vi "Laser Rough Cutting.vi"(0 "configuration file path":path caption="配置文件的路径", 1 "rough cutting msic":T1) -> ()   [LabVIEW 2014]
uses:
  Ctl.xio/rough cutting msic ctl.ctl
  SubVIS.xio/DataSocket/DataSocket_Tags.ctl
  Ctl.xio/part type.ctl
  SubVIS.xio/DataSocket/Write PLC Vars/Write String Var in.vi
  <vilib>/Utility/file.llb/Read From Spreadsheet File (string).vi
  SubVIS.xio/DataSocket/Write PLC Vars/Write Bool Var in.vi
  SubVIS.xio/DataSocket/Read PLC Vars/Read String Var.vi
  SubVIS.xio/DataSocket/Write PLC Vars/Write Dbl Var in.vi
  SubVIS.xio/DataSocket/Read PLC Vars/Read Bool Var.vi
  SubVIS.xio/DataSocket/Read PLC Vars/Read U32 Var.vi
panel:
  in  "SQL information":string
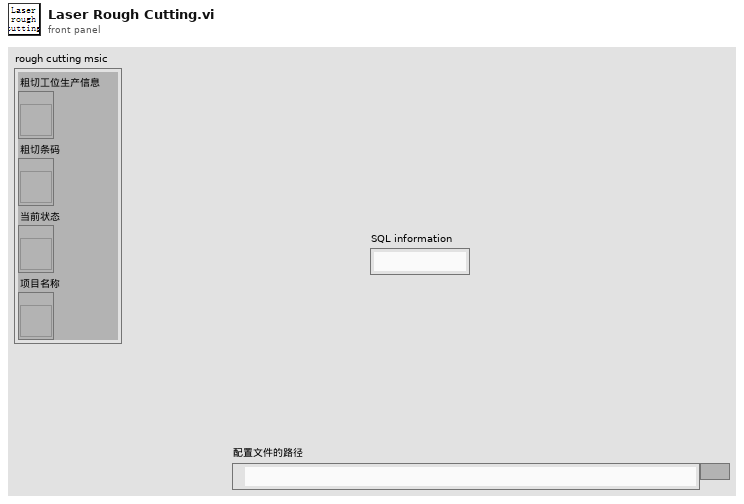
[diagram p1: front panel]
types:
  T1 = cluster{"粗切工位生产信息":refnum<vi>, "粗切条码":refnum<vi>, "当前状态":refnum<vi>, "项目名称":refnum<vi>}
  T2 = typedef "rough cutting msic ctl.ctl" = cluster{"configuration file path":path, "DsOut":T3[], "scanner coms or ip":string, "BarCode":string, "scanner resource name out":refnum<visa-resource-name>, "Hopper car information":cluster{"Hopper car code":string, "Hopper car No":string, "plate No":string}, "pallet.produced number":i32, "SQL information":string, "Database":string[], "Serial number":i32, "database path":path, "rough cutting msic":cluster{"粗切工位生产信息":refnum<vi>, "粗切条码":refnum<vi>, "当前状态":refnum<vi>, "项目名称":refnum<vi>}, "part type":T4, "scanner ip ID":refnum<k5>, "Number of scans ":u8}
  T3 = typedef "DataSocket_Tags.ctl" = cluster{"Ds ID":refnum<k13>, "Tag":string}
  T4 = typedef "part type.ctl" = cluster{"项目号":string, "物料代码":string, "零件号":string, "供应商编码":string, "产线编码":string, "客户代码":string, "颜色代码":string, "托盘上限":i32, "加热温度":string, "加热时长":string, "EOL Stations":string}
  T5 = cluster{"Hopper car code":string, "Hopper car No":string, "plate No":string}
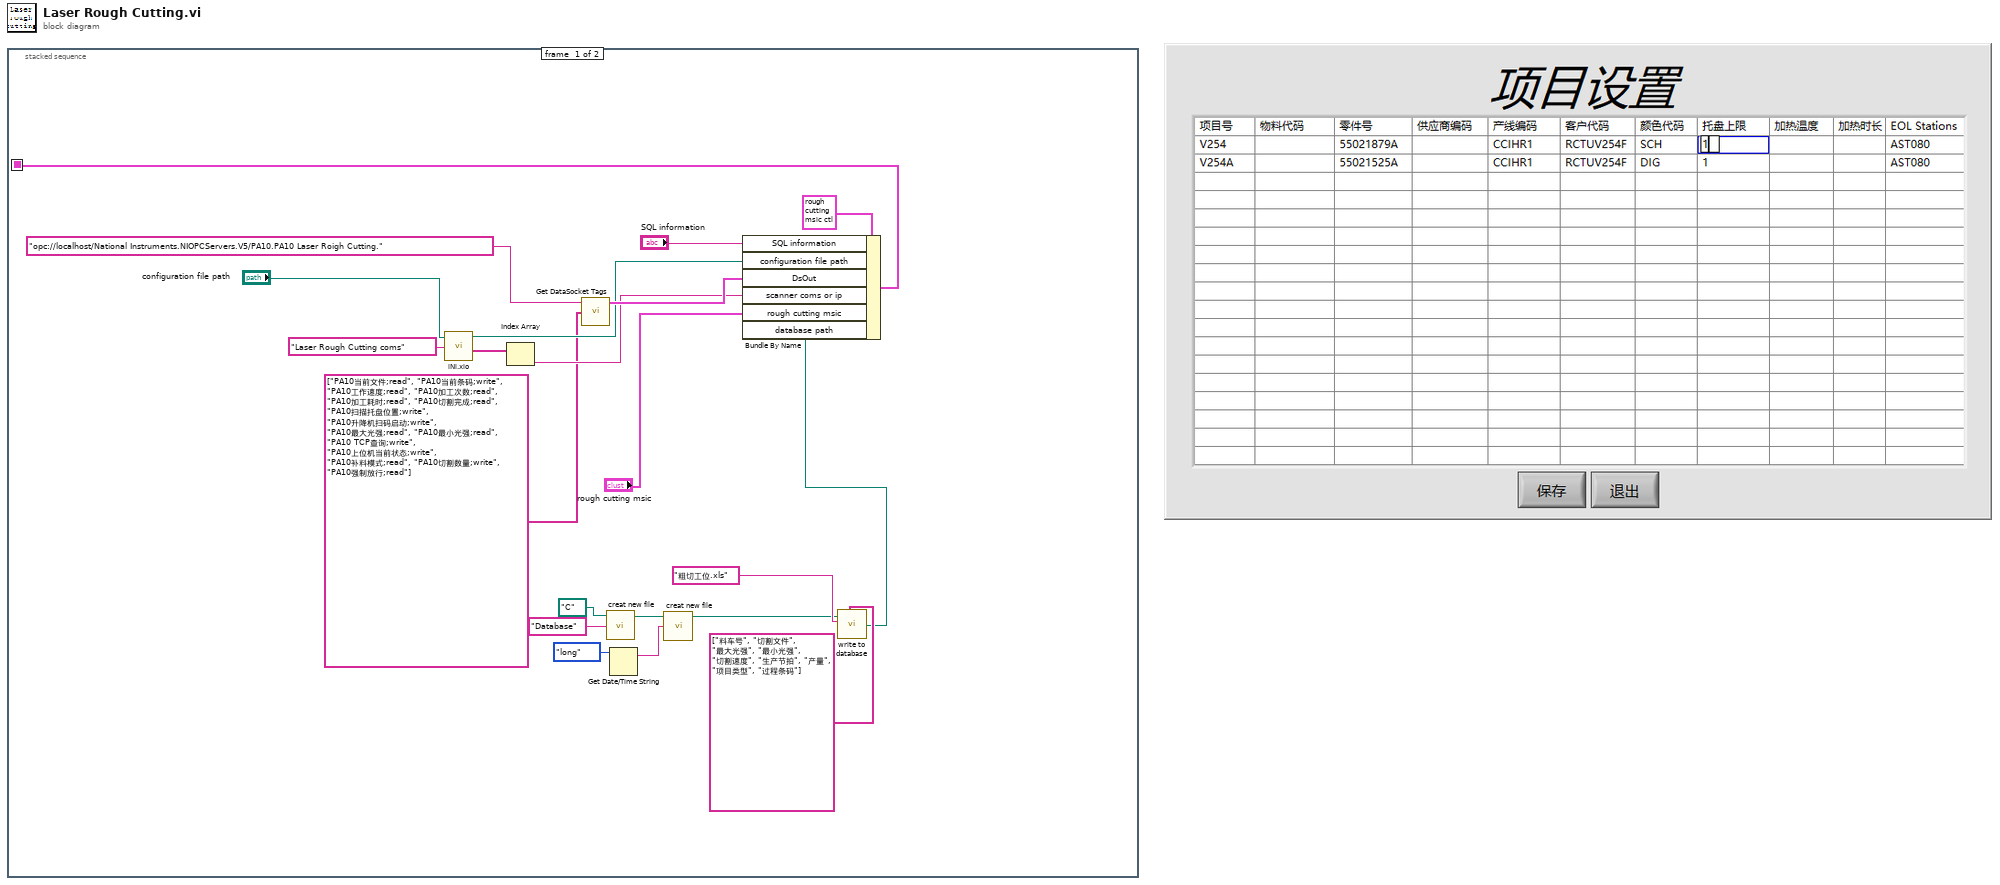
[diagram p0: block diagram]
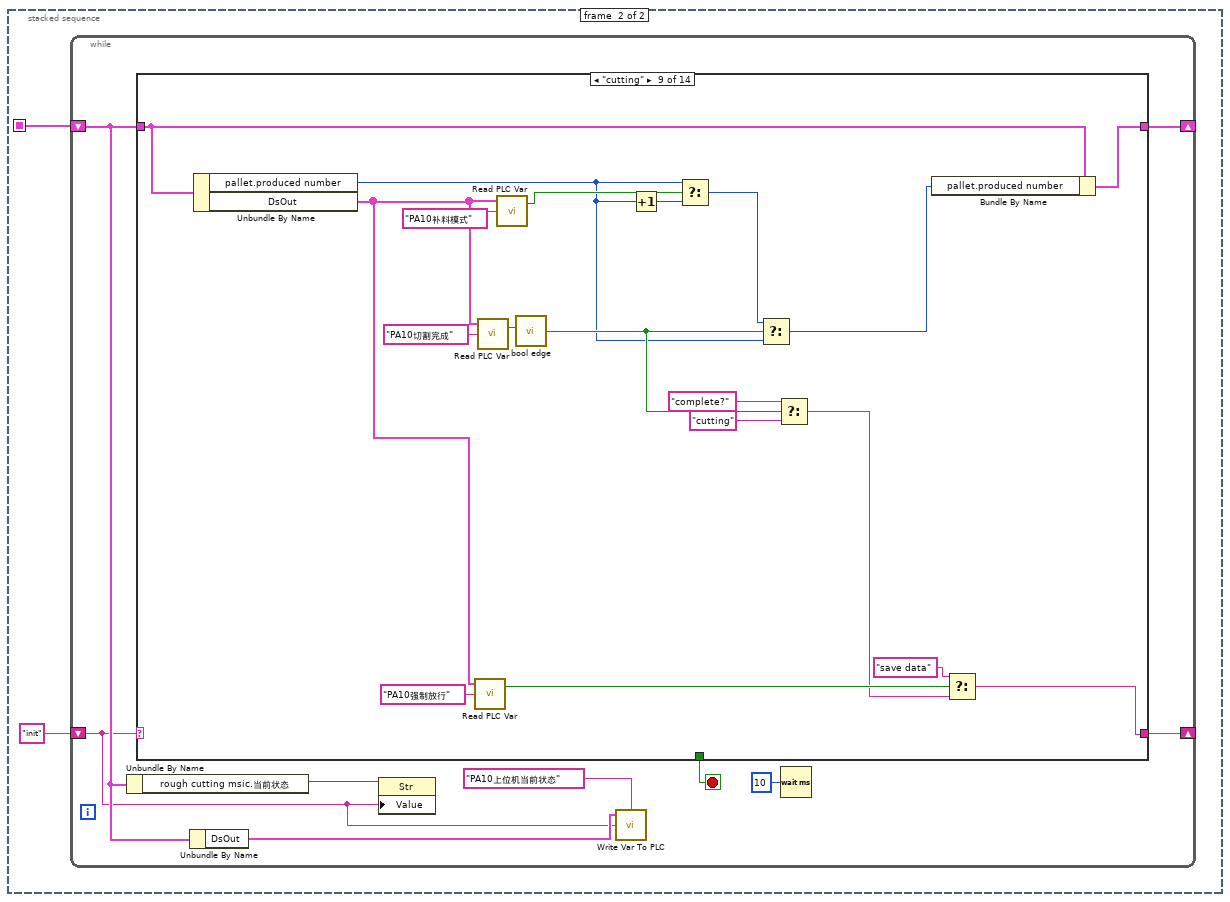
[diagram p2: hidden frame]
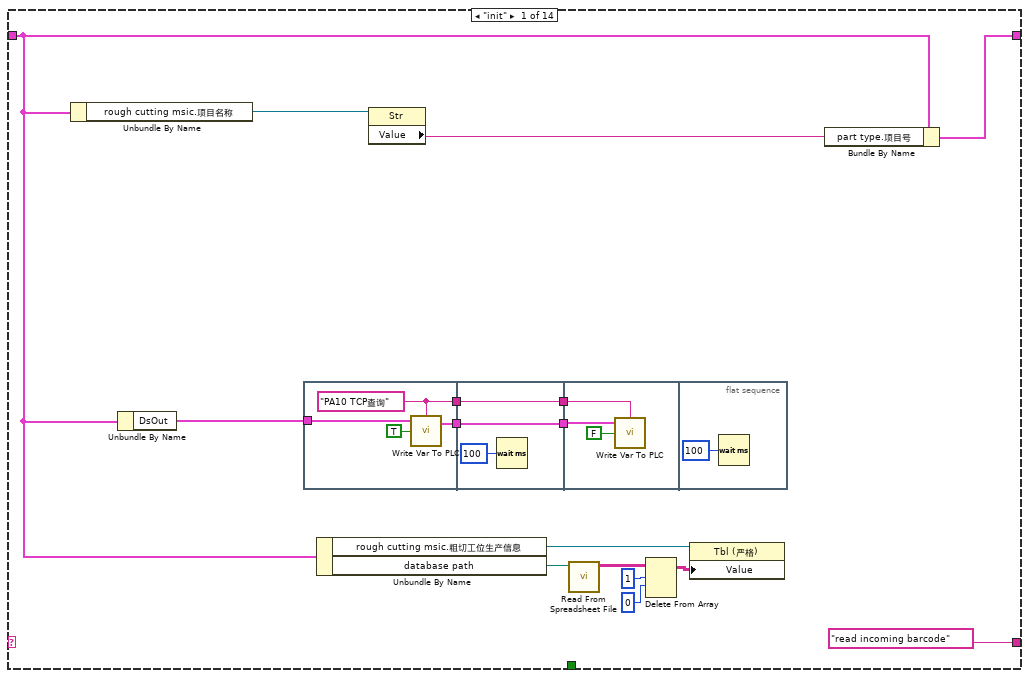
[diagram p3: hidden frame]
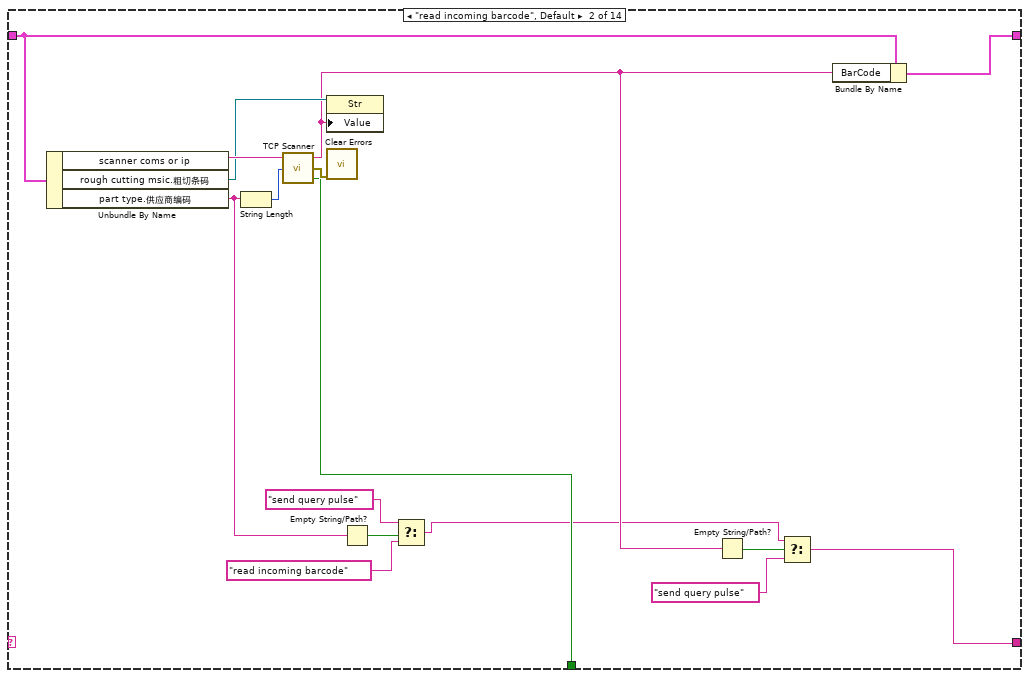
[diagram p4: hidden frame]
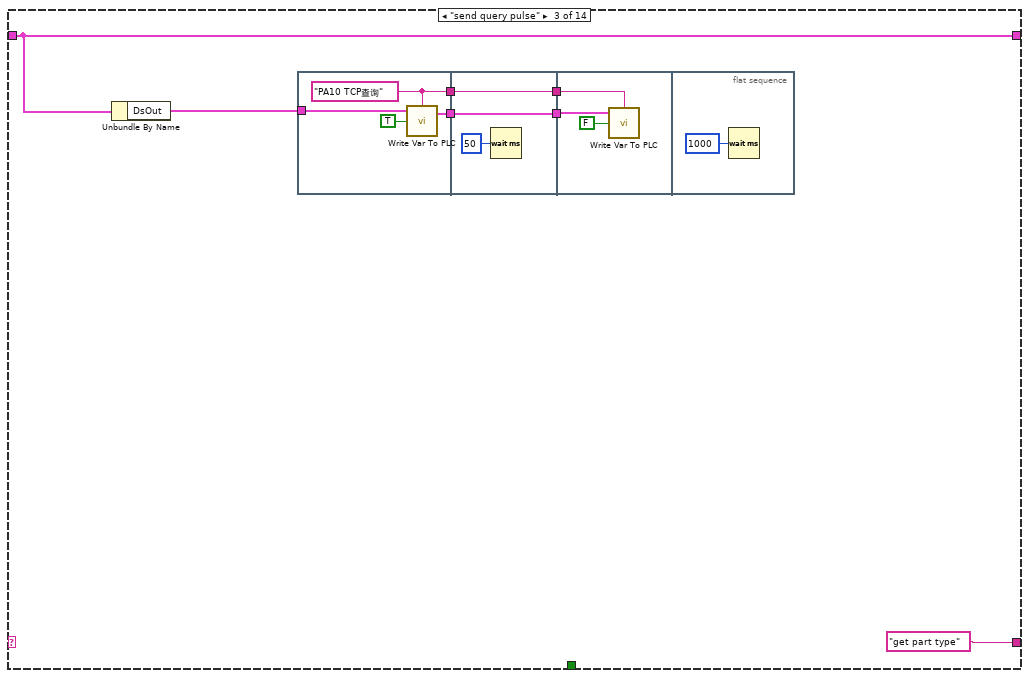
[diagram p5: hidden frame]
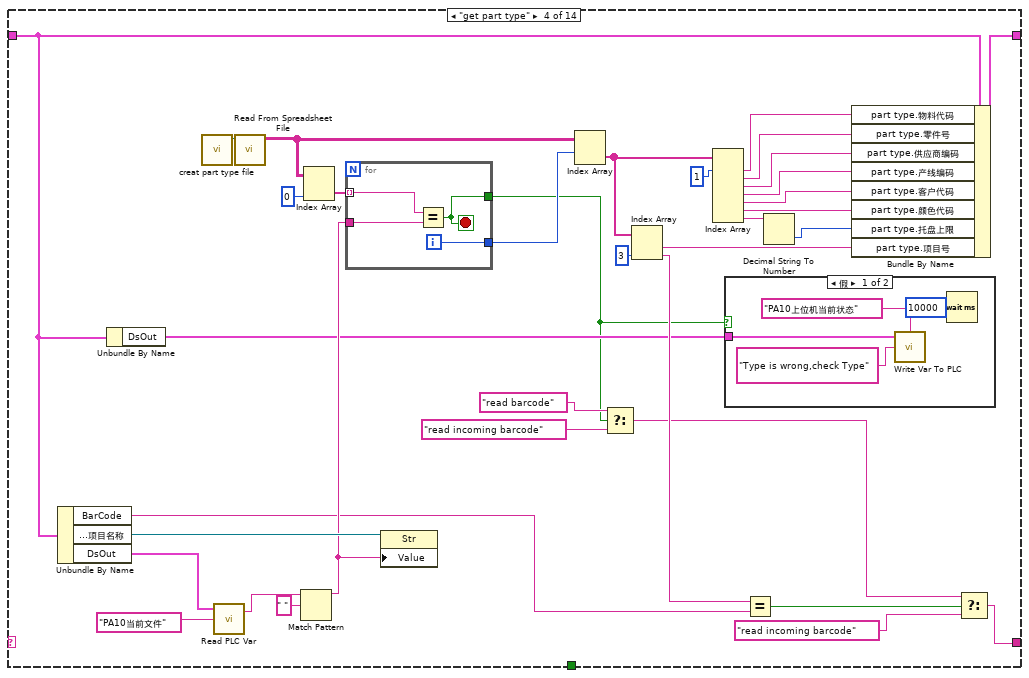
[diagram p6: hidden frame]
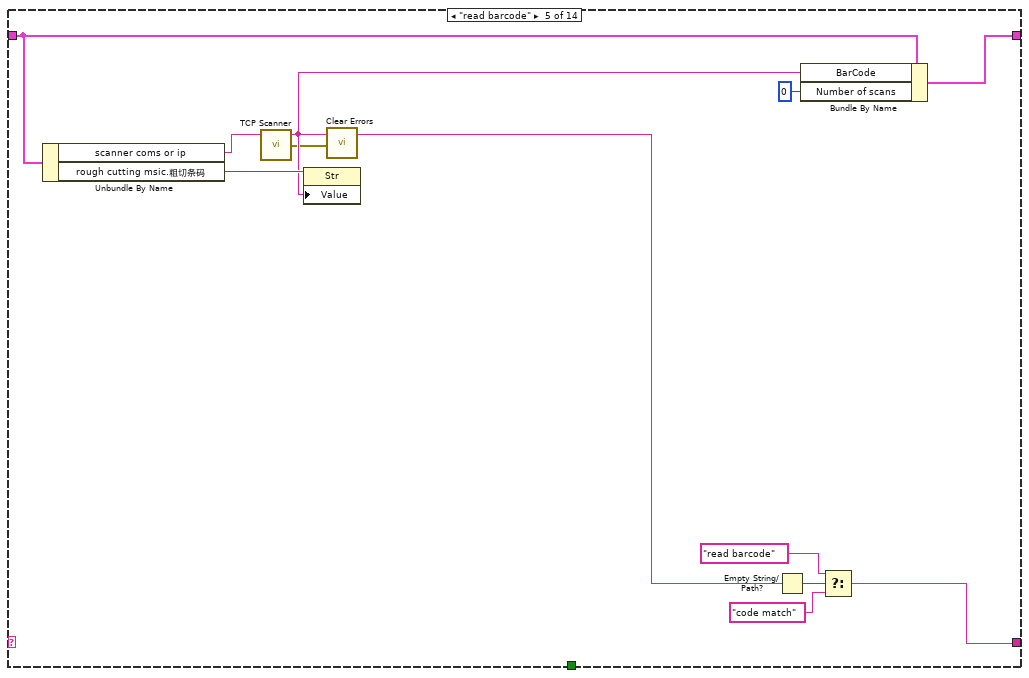
[diagram p8: hidden frame]
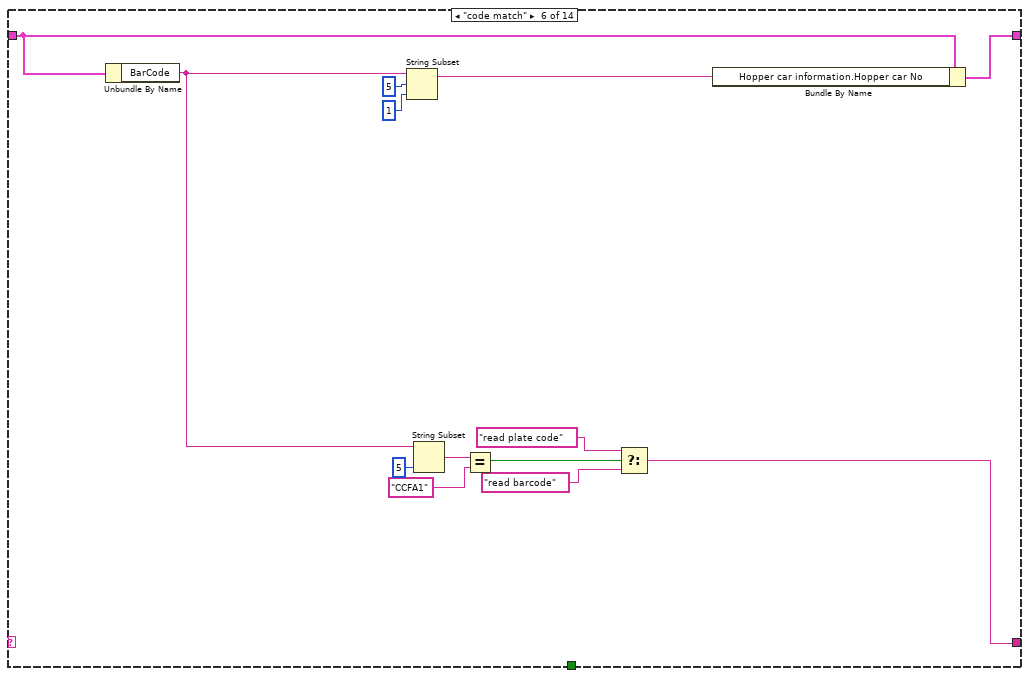
[diagram p9: hidden frame]
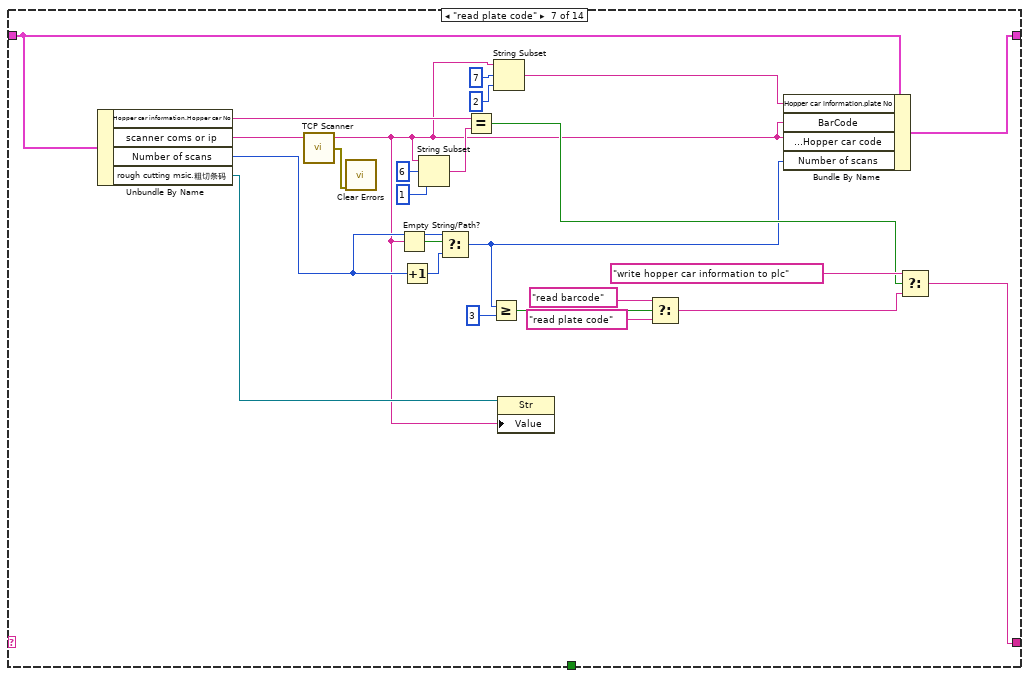
[diagram p10: hidden frame]
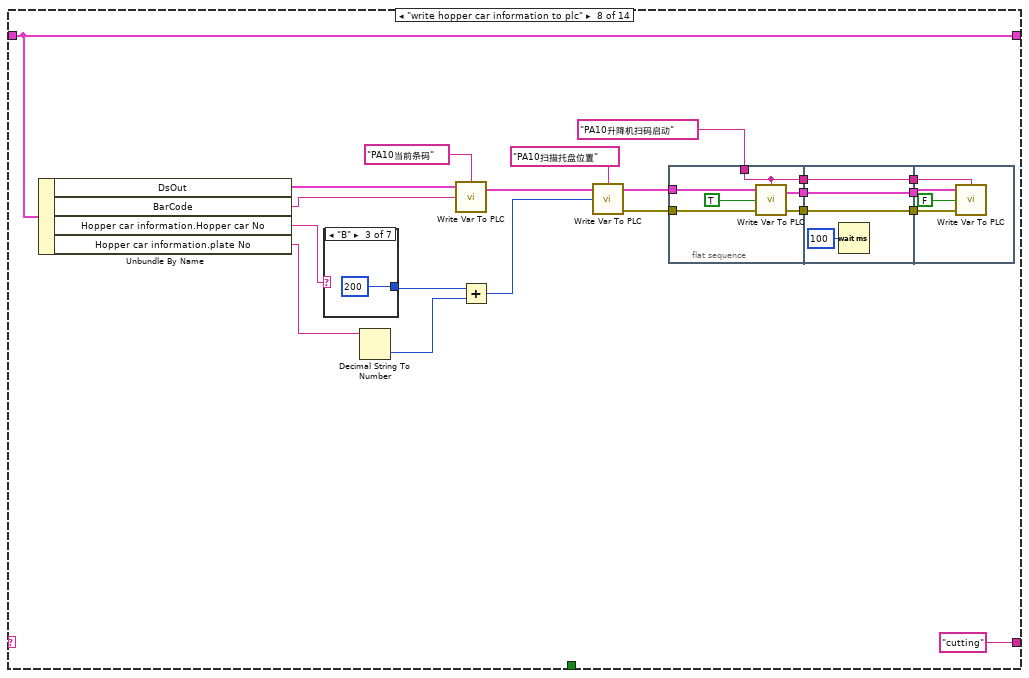
[diagram p11: hidden frame]
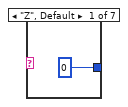
[diagram p12: hidden frame]
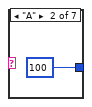
[diagram p13: hidden frame]
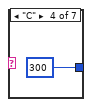
[diagram p14: hidden frame]
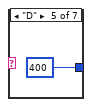
[diagram p15: hidden frame]
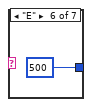
[diagram p16: hidden frame]
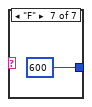
[diagram p17: hidden frame]
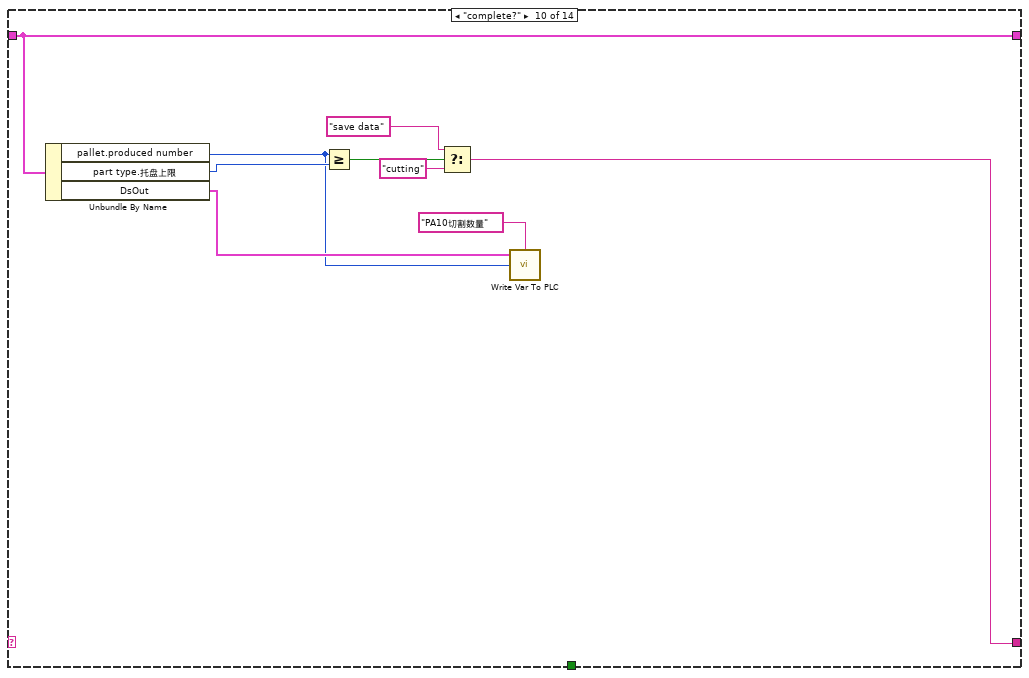
[diagram p18: hidden frame]
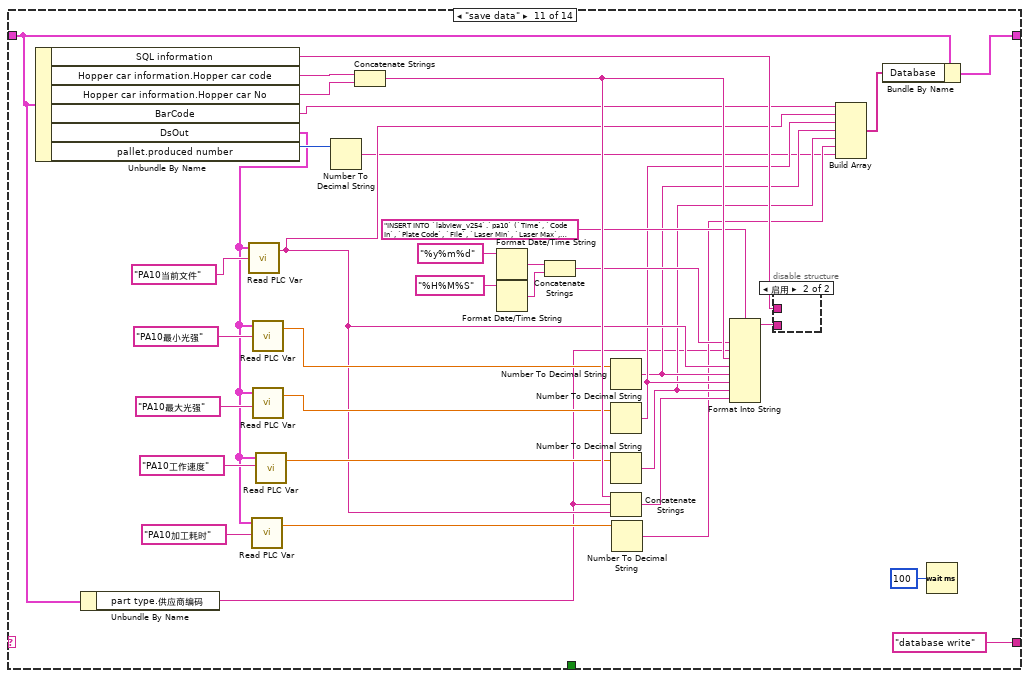
[diagram p19: hidden frame]
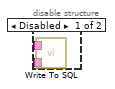
[diagram p20: hidden frame]
diagram:
  n1 = stacked-sequence {
    seq-local: [w10 _] -> [_ w22]
    frame #0 {
      n2 = call "iNi.xio.vi"("configuration file path"="configuration file path", "Sections"="Laser Rough Cutting coms") -> ("configuration file path"=w20:path, "Values"=w18:string[])  [unwired: 1 in, 3 out]
      n3 = Index Array(array=w18) -> (element=w17:string)  [unwired: 1 in]
      n4 = call "Get DataSocket Tags.vi"("All Tags"=string[] ["PA10当前文件;read", "PA10当前条码;write", "PA10工作速度;read", "PA10加工次数;read", "PA10加工耗时;read", "PA10切割完成;read", "PA10扫描托盘位置;write", "PA10升降机扫码启动;write", "PA10最大光强;read", "PA10最小光强;read", "PA10 TCP查询;write", "PA10上位机当前状态;write", "PA10补料模式;read", "PA10切割数量;write", "PA10强制放行;read"], "URL"="opc://localhost/National Instruments.NIOPCServers.V5/PA10.PA10 Laser Roigh Cutting.") -> ("DsOut"=w21:T3[])  [unwired: 3 in]
      n5 = call "creat new file.vi"("file name"="Database", "path"=path "C:/") -> ("created path"=w6:path)  [unwired: 1 in, 2 out]
      n6 = Get Date/Time String(date format (0)=enum16{"short", "long", "abbreviated"}."long" ("日期格式(0)")) -> (date string=w4:string)  [unwired: 2 in, 1 out]
      n7 = call "creat new file.vi"("file name"=w4, "path"=w6) -> ("created path"=w5:path)  [unwired: 1 in, 2 out]
      n8 = call "write to database.vi"("Header"=string[] ["料车号", "切割文件", "最大光强", "最小光强", "切割速度", "生产节拍", "产量", "项目类型", "过程条码"], "file name"="粗切工位.xls", "path"=w5) -> ("new file path (Not A Path if cancelled)"=w1:path)  [unwired: 3 in]
      n9 = Bundle By Name(cluster=T2 {"configuration file path"=path "", "DsOut"=[], "scanner coms or ip"="", "BarCode"="", "scanner resource name out"="", "Hopper car information"={"Hopper car code"="", "Hopper car No"="", "plate No"=""}, "pallet.produced number"=0, "SQL information"="", "Database"=[], "Serial number"=0, "database path"=path "", "rough cutting msic"={"粗切工位生产信息"=refnum, "粗切条码"=refnum, "当前状态"=refnum, "项目名称"=refnum}, "part type"={"项目号"="", "物料代码"="", "零件号"="", "供应商编码"="", "产线编码"="", "客户代码"="", "颜色代码"="", "托盘上限"=0, "加热温度"="", "加热时长"="", "EOL Stations"=""}, "scanner ip ID"=refnum, "Number of scans "=0} ("rough cutting msic"), "SQL information"="SQL information", "configuration file path"=w20, "DsOut"=w21, "scanner coms or ip"=w17, "rough cutting msic"="rough cutting msic", "database path"=w1) -> (w10:T2)
    }
    frame #1 {
      n10 = while {
        shift-right: [w32] -> _
        shift-left: w22 -> [w27]
        shift-right: [w31] -> _
        shift-left: "init" ("event") -> [w25]
        stop <- w24 stop-if-true
        n11 = Unbundle By Name(w27) -> ("rough cutting msic.当前状态"=w29:refnum<vi>)
        n12 = case shown="\"cutting\"" w25 {
          tunnel: w27 -> [w33 w72 w77 w96 w145 w149 w178 w186 w244 w250 w258 w304 w328 w335]
          tunnel: [w48 w75 w77 w128 w144 w157 w177 w186 w246 w250 w263 w316 w328 w340] -> w32
          tunnel: ["read incoming barcode" w66 "get part type" ("f") w121 w140 w155 w180 "cutting" ("event") w229 w253 "database write" ("f") "updata display" ("f") "reset" ("f") "read incoming barcode" ("f")] -> w31
          tunnel: [_ w65 _ _ _ _ _ _ _ _ _ _ _ _] -> w24
          frame "init" {
            n13 = Unbundle By Name(w33) -> ("rough cutting msic.项目名称"=w46:refnum<vi>)
            n14 = Unbundle By Name(w33) -> ("DsOut"=w40:T3[])
            n15 = flat-sequence {
              tunnel: w40 -> [w52]
              tunnel: [w50] -> w44
              tunnel: [w49] -> w43
              tunnel: w44 -> [w54]
              tunnel: [w54] -> w42
              tunnel: w43 -> [w53]
              tunnel: [w53] -> w41
              tunnel: w42 -> [w58]
              tunnel: w41 -> [w56]
              frame #0 {
                w49 = "PA10 TCP查询" ("Tag IN")
                n16 = call-poly "Write Var To PLC.vi"("Tag IN"=w49, "Bool Var in"=TRUE, "Ds PLCTags IN"=w52) -> ("Ds PLCTags OUT"=w50:T3[])  [unwired: 1 in, 1 out]
              }
              frame #1 {
                n17 = Wait (ms)(milliseconds to wait=u32 100 ("等待时间（毫秒）")) -> ()  [unwired: 1 out]
              }
              frame #2 {
                n18 = call-poly "Write Var To PLC.vi"("Tag IN"=w56, "Bool Var in"=FALSE, "Ds PLCTags IN"=w58) -> ()  [unwired: 1 in, 2 out]
              }
              frame #3 {
                n19 = Wait (ms)(milliseconds to wait=u32 100 ("等待时间（毫秒）")) -> ()  [unwired: 1 out]
              }
            }
            n20 = Unbundle By Name(w33) -> ("rough cutting msic.粗切工位生产信息"=w39:refnum<vi>, "database path"=w38:path)
            n21 = property class="Str"(reference=w46) -> ("Value"=w45:string)  [unwired: 1 in, 2 out]
            n22 = call-poly <vilib>:"Read From Spreadsheet File.vi"("file path (dialog if empty)"=w38) -> ("all rows"=w37:string[][])  [unwired: 6 in, 4 out]
            n23 = Delete From Array(array=w37, length=1 ("长度"), index (row)=0 ("索引 (行)")) -> (array with subset deleted=w34:string[][])  [unwired: 1 in, 1 out]
            n24 = property class="Tbl (严格)"(reference=w39, "Value"=w34) -> ()  [unwired: 1 in, 2 out]
            n25 = Bundle By Name(cluster=w33, "part type.项目号"=w45) -> (w48:T2)
          }
          frame "read incoming barcode", Default {
            n26 = Unbundle By Name(w72) -> ("scanner coms or ip"=w74:string, "rough cutting msic.粗切条码"=w73:refnum<vi>, "part type.供应商编码"=w63:string)
            n27 = String Length(string=w63) -> (length=w71:i32)
            n28 = call "TCP Scanner.vi"("byte of read(9)"=w71, "ip"=w74) -> ("status"=w65:bool, "错误输出"=w70:errorcluster, "Barcode"=w69:string)  [unwired: 1 in]
            n29 = property class="Str"(reference=w73, "Value"=w69) -> ()  [unwired: 1 in, 2 out]
            n30 = call <vilib>:"Clear Errors.vi"("error in (no error)"=w70) -> ()  [unwired: 5 in, 2 out]
            n31 = Empty String/Path?(string/path=w63) -> (empty?=w64:bool)
            n32 = Select(t="send query pulse" ("f"), s=w64, f="read incoming barcode") -> (s? t:f=w60:string)
            n33 = Empty String/Path?(string/path=w69) -> (empty?=w68:bool)
            n34 = Select(t=w60, s=w68, f="send query pulse") -> (s? t:f=w66:string)
            n35 = Bundle By Name(cluster=w72, "BarCode"=w69) -> (w75:T2)
          }
          frame "send query pulse" {
            n36 = Unbundle By Name(w77) -> ("DsOut"=w78:T3[])
            n37 = flat-sequence {
              tunnel: w78 -> [w86]
              tunnel: [w84] -> w82
              tunnel: [w83] -> w81
              tunnel: w82 -> [w88]
              tunnel: [w88] -> w80
              tunnel: w81 -> [w87]
              tunnel: [w87] -> w79
              tunnel: w80 -> [w92]
              tunnel: w79 -> [w90]
              frame #0 {
                w83 = "PA10 TCP查询" ("Tag IN")
                n38 = call-poly "Write Var To PLC.vi"("Tag IN"=w83, "Bool Var in"=TRUE, "Ds PLCTags IN"=w86) -> ("Ds PLCTags OUT"=w84:T3[])  [unwired: 1 in, 1 out]
              }
              frame #1 {
                n39 = Wait (ms)(milliseconds to wait=u32 50 ("等待时间（毫秒）")) -> ()  [unwired: 1 out]
              }
              frame #2 {
                n40 = call-poly "Write Var To PLC.vi"("Tag IN"=w90, "Bool Var in"=FALSE, "Ds PLCTags IN"=w92) -> ()  [unwired: 1 in, 2 out]
              }
              frame #3 {
                n41 = Wait (ms)(milliseconds to wait=u32 1000 ("等待时间（毫秒）")) -> ()  [unwired: 1 out]
              }
            }
          }
          frame "get part type" {
            n42 = Unbundle By Name(w96) -> ("BarCode"=w102:string, "rough cutting msic.项目名称"=w104:refnum<vi>, "DsOut"=w111:T3[])
            n43 = Unbundle By Name(w96) -> ("DsOut"=w95:T3[])
            n44 = call "creat part type file.vi"() -> ("new file path (Not A Path if cancelled)"=w122:path)  [unwired: 11 in]
            n45 = call-poly "Read PLC Var.vi"("Tag IN"="PA10当前文件", "Ds PLCTags IN"=w111) -> ("String Var out"=w106:string)  [unwired: 1 in, 1 out]
            n46 = call-poly <vilib>:"Read From Spreadsheet File.vi"("file path (dialog if empty)"=w122) -> ("all rows"=w124:string[][])  [unwired: 6 in, 4 out]
            n47 = Match Pattern(string=w106, regular expression=" " ("正则表达式")) -> (before substring=w103:string)  [unwired: 1 in, 3 out]
            n48 = Index Array(array=w124, index (col)=0 ("禁用的索引 (列)")) -> (element=w125:string[])  [unwired: 1 in]
            n49 = for {
              tunnel: w125 -> [w134] mode=indexing
              tunnel: [w136] -> w123
              tunnel: w103 -> [w135]
              tunnel: [w133] -> w94
              i -> [w136]
              stop <- w133 stop-if-true
              n50 = Equal?(x=w134, y=w135) -> (x = y?=w133:bool)
            }
            n51 = property class="Str"(reference=w104, "Value"=w103) -> ()  [unwired: 1 in, 2 out]
            n52 = Index Array(array=w124, index (row)=w123) -> (element=w110:string[])  [unwired: 1 in]
            n53 = Select(t="read barcode", s=w94, f="read incoming barcode") -> (s? t:f=w97:string)
            n54 = Index Array(array=w110, index #2=3 ("索引")) -> (element #1=w108:string, element #2=w101:string)  [unwired: 1 in]
            n55 = Index Array(array=w110, index #1=1 ("索引")) -> (element #1=w119:string, element #2=w118:string, element #3=w117:string, element #4=w116:string, element #5=w115:string, element #6=w114:string, element #7=w113:string)  [unwired: 6 in]
            n56 = case shown="假" w94 {
              tunnel: w95 -> [w132 _]
              frame False {
                n57 = call-poly "Write Var To PLC.vi"("Tag IN"="PA10上位机当前状态", "String Var in"="Type is wrong,check Type", "Ds PLCTags IN"=w132) -> ()  [unwired: 1 in, 2 out]
                n58 = Wait (ms)(milliseconds to wait=u32 10000 ("等待时间（毫秒）")) -> ()  [unwired: 1 out]
              }
              frame True {
              }
            }
            n59 = Equal?(x=w101, y=w102) -> (x = y?=w109:bool)
            n60 = Decimal String To Number(string=w113) -> (number=w120:i32)  [unwired: 2 in, 1 out]
            n61 = Bundle By Name(cluster=w96, "part type.物料代码"=w119, "part type.零件号"=w118, "part type.供应商编码"=w117, "part type.产线编码"=w116, "part type.客户代码"=w115, "part type.颜色代码"=w114, "part type.托盘上限"=w120, "part type.项目号"=w108) -> (w128:T2)
            n62 = Select(t=w97, s=w109, f="read incoming barcode") -> (s? t:f=w121:string)
          }
          frame "read barcode" {
            n63 = Unbundle By Name(w145) -> ("scanner coms or ip"=w147:string, "rough cutting msic.粗切条码"=w146:refnum<vi>)
            n64 = call "TCP Scanner.vi"("ip"=w147) -> ("错误输出"=w138:errorcluster, "Barcode"=w139:string)  [unwired: 2 in, 1 out]
            n65 = property class="Str"(reference=w146, "Value"=w139) -> ()  [unwired: 1 in, 2 out]
            n66 = call <vilib>:"Clear Errors.vi"("error in (no error)"=w138) -> ()  [unwired: 5 in, 2 out]
            n67 = Empty String/Path?(string/path=w139) -> (empty?=w143:bool)
            n68 = Bundle By Name(cluster=w145, "BarCode"=w139, "Number of scans"=u8 0) -> (w144:T2)
            n69 = Select(t="read barcode", s=w143, f="code match") -> (s? t:f=w140:string)
          }
          frame "code match" {
            n70 = Unbundle By Name(w149) -> ("BarCode"=w148:string)
            n71 = String Subset(string=w148, offset (0)=5 ("偏移量(0)"), length (rest)=1 ("长度（剩余）")) -> (substring=w151:string)
            n72 = String Subset(string=w148, length (rest)=5 ("长度（剩余）")) -> (substring=w152:string)  [unwired: 1 in]
            n73 = Equal?(x=w152, y="CCFA1") -> (x = y?=w156:bool)
            n74 = Select(t="read plate code" ("event"), s=w156, f="read barcode" ("event")) -> (s? t:f=w155:string)
            n75 = Bundle By Name(cluster=w149, "Hopper car information.Hopper car No"=w151) -> (w157:T2)
          }
          frame "read plate code" {
            n76 = Unbundle By Name(w178) -> ("Hopper car information.Hopper car No"=w182:string, "scanner coms or ip"=w185:string, "Number of scans"=w168:u8, "rough cutting msic.粗切条码"=w165:refnum<vi>)
            n77 = call "TCP Scanner.vi"("ip"=w185) -> ("错误输出"=w170:errorcluster, "Barcode"=w162:string)  [unwired: 2 in, 1 out]
            n78 = call <vilib>:"Clear Errors.vi"("error in (no error)"=w170) -> ()  [unwired: 5 in, 2 out]
            n79 = Empty String/Path?(string/path=w162) -> (empty?=w169:bool)
            n80 = Increment(x=w168) -> (x+1=w167:u8)
            n81 = String Subset(string=w162, offset (0)=6 ("偏移量(0)"), length (rest)=1 ("长度（剩余）")) -> (substring=w176:string)
            n82 = Select(t=w168, s=w169, f=w167) -> (s? t:f=w166:u8)
            n83 = Equal?(x=w182, y=w176) -> (x = y?=w179:bool)
            n84 = Greater Or Equal?(x=w166, y=u8 3) -> (x >= y?=w174:bool)
            n85 = String Subset(string=w162, offset (0)=7 ("偏移量(0)"), length (rest)=2 ("长度（剩余）")) -> (substring=w161:string)
            n86 = property class="Str"(reference=w165, "Value"=w162) -> ()  [unwired: 1 in, 2 out]
            n87 = Select(t="read barcode" ("event"), s=w174, f="read plate code" ("event")) -> (s? t:f=w171:string)
            n88 = Bundle By Name(cluster=w178, "Hopper car information.plate No"=w161, "BarCode"=w162, "Hopper car information.Hopper car code"=w162, "Number of scans"=w166) -> (w177:T2)
            n89 = Select(t="write hopper car information to plc" ("event"), s=w179, f=w171) -> (s? t:f=w180:string)
          }
          frame "write hopper car information to plc" {
            n90 = Unbundle By Name(w186) -> ("DsOut"=w189:T3[], "BarCode"=w188:string, "Hopper car information.Hopper car No"=w206:string, "Hopper car information.plate No"=w205:string)
            n91 = case shown="\"B\"" w206 {
              tunnel: [0 100 200 300 400 500 600] -> w204
              frame "Z", Default {
              }
              frame "A" {
              }
              frame "B" {
              }
              frame "C" {
              }
              frame "D" {
              }
              frame "E" {
              }
              frame "F" {
              }
            }
            n92 = Decimal String To Number(string=w205) -> (number=w203:i32)  [unwired: 2 in, 1 out]
            n93 = call-poly "Write Var To PLC.vi"("Tag IN"="PA10当前条码", "String Var in"=w188, "Ds PLCTags IN"=w189) -> ("Ds PLCTags OUT"=w190:T3[])  [unwired: 1 in, 1 out]
            n94 = Add(x=w204, y=w203) -> (x+y=w201:i32)
            n95 = call-poly "Write Var To PLC.vi"("Tag IN"="PA10扫描托盘位置", "Dbl Var in"=w201, "Ds PLCTags IN"=w190) -> ("error out"=w200:errorcluster, "Ds PLCTags OUT"=w199:T3[])  [unwired: 1 in]
            n96 = flat-sequence {
              tunnel: w200 -> [w212]
              tunnel: w199 -> [w211]
              tunnel: "PA10升降机扫码启动" ("Tag IN") -> [w208]
              tunnel: [w209] -> w195
              tunnel: [w208] -> w194
              tunnel: [w207] -> w192
              tunnel: [w215] -> w196
              tunnel: w195 -> [w215]
              tunnel: w194 -> [w214]
              tunnel: [w214] -> w193
              tunnel: w192 -> [w213]
              tunnel: [w213] -> w191
              tunnel: w196 -> [w220]
              tunnel: w193 -> [w219]
              tunnel: w191 -> [w218]
              frame #0 {
                n97 = call-poly "Write Var To PLC.vi"("Tag IN"=w208, "错误输入（无错误）"=w212, "Bool Var in"=TRUE, "Ds PLCTags IN"=w211) -> ("error out"=w207:errorcluster, "Ds PLCTags OUT"=w209:T3[])
              }
              frame #1 {
                n98 = Wait (ms)(milliseconds to wait=u32 100 ("等待时间（毫秒）")) -> ()  [unwired: 1 out]
              }
              frame #2 {
                n99 = call-poly "Write Var To PLC.vi"("Tag IN"=w219, "错误输入（无错误）"=w218, "Bool Var in"=FALSE, "Ds PLCTags IN"=w220) -> ()  [unwired: 2 out]
              }
            }
          }
          frame "cutting" {
            n100 = Unbundle By Name(w244) -> ("pallet.produced number"=w235:i32, "DsOut"=w232:T3[])
            n101 = call-poly "Read PLC Var.vi"("Tag IN"="PA10强制放行", "Ds PLCTags IN"=w232) -> ("Bool Var out"=w231:bool)  [unwired: 1 in, 1 out]
            n102 = call-poly "Read PLC Var.vi"("Tag IN"="PA10切割完成", "Ds PLCTags IN"=w232) -> ("Bool Var out"=w239:bool)  [unwired: 1 in, 1 out]
            n103 = call-poly "Read PLC Var.vi"("Tag IN"="PA10补料模式", "Ds PLCTags IN"=w232) -> ("Bool Var out"=w237:bool)  [unwired: 1 in, 1 out]
            n104 = call "bool edge.vi"("bool in"=w239) -> ("true-false"=w243:bool)  [unwired: 6 in, 1 out]
            n105 = Increment(x=w235) -> (x+1=w236:i32)
            n106 = Select(t=w235, s=w237, f=w236) -> (s? t:f=w234:i32)
            n107 = Select(t=w234, s=w243, f=w235) -> (s? t:f=w245:i32)
            n108 = Select(t="complete?" ("event"), s=w243, f="cutting" ("event")) -> (s? t:f=w230:string)
            n109 = Bundle By Name(cluster=w244, "pallet.produced number"=w245) -> (w246:T2)
            n110 = Select(t="save data" ("event"), s=w231, f=w230) -> (s? t:f=w229:string)
          }
          frame "complete?" {
            n111 = Unbundle By Name(w250) -> ("pallet.produced number"=w248:i32, "part type.托盘上限"=w255:i32, "DsOut"=w249:T3[])
            n112 = Greater Or Equal?(x=w248, y=w255) -> (x >= y?=w254:bool)
            n113 = Select(t="save data" ("event"), s=w254, f="cutting") -> (s? t:f=w253:string)
            n114 = call-poly "Write Var To PLC.vi"("Tag IN"="PA10切割数量", "Dbl Var in"=w248, "Ds PLCTags IN"=w249) -> ()  [unwired: 1 in, 2 out]
          }
          frame "save data" {
            n115 = Unbundle By Name(w258) -> ("SQL information"=w273:string, "Hopper car information.Hopper car code"=w275:string, "Hopper car information.Hopper car No"=w274:string, "BarCode"=w260:string, "DsOut"=w259:T3[], "pallet.produced number"=w262:i32)
            n116 = Unbundle By Name(w258) -> ("part type.供应商编码"=w257:string)
            n117 = call-poly "Read PLC Var.vi"("Tag IN"="PA10当前文件", "Ds PLCTags IN"=w259) -> ("String Var out"=w271:string)  [unwired: 1 in, 1 out]
            n118 = call-poly "Read PLC Var.vi"("Tag IN"="PA10加工耗时", "Ds PLCTags IN"=w259) -> ("U32 Var out"=w266:dbl)  [unwired: 1 in, 1 out]
            n119 = call-poly "Read PLC Var.vi"("Tag IN"="PA10最小光强", "Ds PLCTags IN"=w259) -> ("U32 Var out"=w280:dbl)  [unwired: 1 in, 1 out]
            n120 = call-poly "Read PLC Var.vi"("Tag IN"="PA10最大光强", "Ds PLCTags IN"=w259) -> ("U32 Var out"=w278:dbl)  [unwired: 1 in, 1 out]
            n121 = call-poly "Read PLC Var.vi"("Tag IN"="PA10工作速度", "Ds PLCTags IN"=w259) -> ("U32 Var out"=w276:dbl)  [unwired: 1 in, 1 out]
            n122 = Number To Decimal String(number=w262) -> (decimal integer string=w261:string)  [unwired: 1 in]
            n123 = Concatenate Strings(w275, w274) -> (w291:string)
            n124 = Format Date/Time String(time format string (%c)="%y%m%d" ("时间格式字符串(%c)")) -> (date/time string=w286:string)  [unwired: 2 in]
            n125 = Format Date/Time String(time format string (%c)="%H%M%S" ("时间格式字符串(%c)")) -> (date/time string=w285:string)  [unwired: 2 in]
            n126 = Concatenate Strings(w286, w285) -> (w283:string)
            n127 = Number To Decimal String(number=w280) -> (decimal integer string=w269:string)  [unwired: 1 in]
            n128 = Number To Decimal String(number=w278) -> (decimal integer string=w270:string)  [unwired: 1 in]
            n129 = Number To Decimal String(number=w276) -> (decimal integer string=w268:string)  [unwired: 1 in]
            n130 = Concatenate Strings(w291, w257, w271) -> (w288:string)
            n131 = Number To Decimal String(number=w266) -> (decimal integer string=w265:string)  [unwired: 1 in]
            n132 = Format Into String(format string="INSERT INTO `labview_v254`.`pa10` (`Time`, `Code In`, `Plate Code`, `File`, `Laser Min`, `Laser Max`, `Vel`, `Code Out`) VALUES ('%s', '%s', '%s', '%s', '%s', '%s', '%s', '%s');", w283, w257, w291, w271, w269, w270, w268, w288) -> (resulting string=w289:string)  [unwired: 2 in, 1 out]
            n133 = disable-structure shown="启用" {
              disable-tunnel: w289 -> [w293 _]
              disable-tunnel: w273 -> [w292 _]
              frame Disabled {
                n134 = call "Write To SQL.vi"("SQL query"=w293, "connection information"=w292) -> ()  [unwired: 1 out]
              }
              frame Enabled {
              }
            }
            n135 = Build Array(w260, w271, w270, w269, w268, w265, w261) -> (w264:string[])
            n136 = Bundle By Name(cluster=w258, "Database"=w264) -> (w263:T2)
            n137 = Wait (ms)(milliseconds to wait=u32 100 ("等待时间（毫秒）")) -> ()  [unwired: 1 out]
          }
          frame "database write" {
            w301 = enum16{"read", "write"}."write" ("write\\read")
            n138 = Unbundle By Name(w304) -> ("configuration file path"=w303:path, "BarCode"=w300:string)
            n139 = Unbundle By Name(w304) -> ("Database"=w311:string[], "part type.项目号"=w309:string, "Hopper car information.Hopper car code"=w308:string)
            n140 = Get Date/Time In Seconds() -> (seconds since 1Jan1904=w307:timestamp)
            n141 = Format Date/Time String(time format string (%c)="%y%m%d%H%M" ("时间格式字符串(%c)"), seconds (now)=w307) -> (date/time string=w305:string)  [unwired: 1 in]
            n142 = Concatenate Strings(w309, w308, w305) -> (w296:string)
            n143 = String Subset(string=w300, length (rest)=6 ("长度（剩余）")) -> (substring=w298:string)  [unwired: 1 in]
            n144 = call "Hopper car inf.vi"("write\\read（read)"=w301, "value"=w296, "key"=w300, "path in"=w303) -> ("path out"=w302:path)  [unwired: 6 in, 1 out]
            n145 = Build Array (concatenate)(w311, w309, w296) -> (w310:string[])
            n146 = Concatenate Strings(w298, "000") -> (w295:string)
            n147 = call "Hopper car inf.vi"("write\\read（read)"=w301, "value"=w296, "key"=w295, "path in"=w302) -> ()  [unwired: 6 in, 2 out]
            n148 = call "creat new file.vi"("file name"="Database", "path"=path "C:/") -> ("created path"=w315:path)  [unwired: 1 in, 2 out]
            n149 = Get Date/Time String(date format (0)=enum16{"short", "long", "abbreviated"}."long" ("日期格式(0)")) -> (date string=w313:string)  [unwired: 2 in, 1 out]
            n150 = call "creat new file.vi"("file name"=w313, "path"=w315) -> ("created path"=w314:path)  [unwired: 1 in, 2 out]
            n151 = call "write to database.vi"("Header"=string[] ["料车号", "切割文件", "最大光强", "最小光强", "切割速度", "生产节拍", "产量", "项目类型", "过程条码"], "data in"=w310, "file name"="粗切工位.xls", "path"=w314) -> ("new file path (Not A Path if cancelled)"=w317:path)  [unwired: 2 in]
            n152 = Bundle By Name(cluster=w304, "database path"=w317) -> (w316:T2)
            n153 = Wait (ms)(milliseconds to wait=u32 100 ("等待时间（毫秒）")) -> ()  [unwired: 1 out]
          }
          frame "updata display" {
            n154 = Unbundle By Name(w328) -> ("rough cutting msic.粗切工位生产信息"=w330:refnum<vi>, "database path"=w329:path)
            n155 = call-poly <vilib>:"Read From Spreadsheet File.vi"("file path (dialog if empty)"=w329) -> ("all rows"=w327:string[][])  [unwired: 6 in, 4 out]
            n156 = Delete From Array(array=w327, length=1 ("长度"), index (row)=0 ("索引 (行)")) -> (array with subset deleted=w324:string[][])  [unwired: 1 in, 1 out]
            n157 = property class="Tbl (严格)"(reference=w330, "Value"=w324) -> ()  [unwired: 1 in, 2 out]
            n158 = Wait (ms)(milliseconds to wait=u32 100 ("等待时间（毫秒）")) -> ()  [unwired: 1 out]
          }
          frame "reset" {
            n159 = Unbundle By Name(w335) -> ("rough cutting msic.粗切条码"=w334:refnum<vi>)
            n160 = property class="Str"(reference=w334, "Value"="" ("值")) -> ()  [unwired: 1 in, 2 out]
            n161 = Bundle By Name(cluster=w335, "Number of scans"=u8 0, "pallet.produced number"=0, "BarCode"="", "Database"=string[] [], "Hopper car information"=T5 {"Hopper car code"="", "Hopper car No"="", "plate No"=""}) -> (w340:T2)
            n162 = Wait (ms)(milliseconds to wait=u32 100 ("等待时间（毫秒）")) -> ()  [unwired: 1 out]
          }
        }
        n163 = Unbundle By Name(w27) -> ("DsOut"=w26:T3[])
        n164 = property class="Str"(reference=w29, "Value"=w25) -> ()  [unwired: 1 in, 2 out]
        n165 = call-poly "Write Var To PLC.vi"("Tag IN"="PA10上位机当前状态", "String Var in"=w25, "Ds PLCTags IN"=w26) -> ()  [unwired: 1 in, 2 out]
        n166 = Wait (ms)(milliseconds to wait=u32 10 ("等待时间（毫秒）")) -> ()  [unwired: 1 out]
      }
    }
  }
